vi "check_amp_mio.vi"() -> ()   [LabVIEW 2013]
uses:
  <vilib>/DAQmx/write.llb/DAQmx Write (Digital Bool 1Line 1Point).vi
  <vilib>/DAQmx/create/channels.llb/DAQmx Create Channel (DO-Digital Output).vi
  <vilib>/DAQmx/miscellaneous.llb/DAQmx Fill In Error Info.vi
panel:
  in  "data":bool
  in  "lines":tag
  in  "Exit":bool
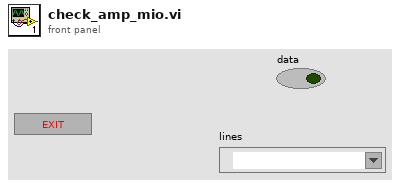
[diagram p1: front panel]
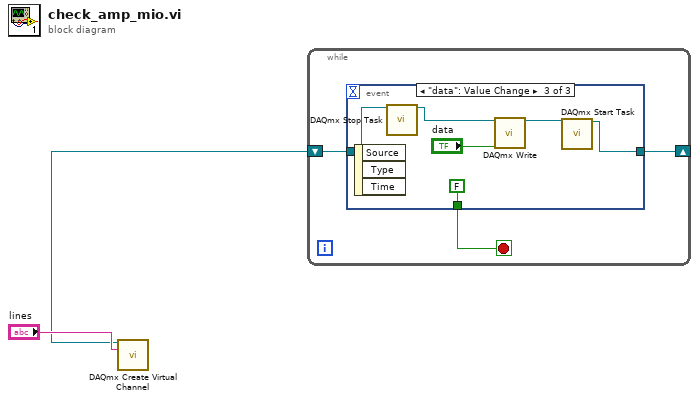
[diagram p0: block diagram]
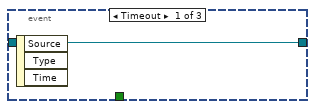
[diagram p2: hidden frame]
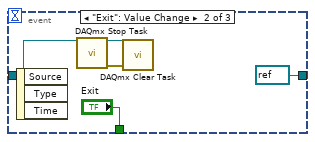
[diagram p3: hidden frame]
diagram:
  n1 = call-poly <vilib>:"DAQmx Create Virtual Channel.vi"("lines"="lines") -> ("task out"=w1:refnum<k21>)  [unwired: 13 in, 1 out]
  n2 = while {
    shift-right: [w3] -> _
    shift-left: w1 -> [w5]
    stop <- w4 stop-if-true
    n3 = event shown="[2] \"data\": Value Change" {
      selector: _ -> [_ _ _]
      dyn-events: _ -> [_ _ _]
      timeout: _ -> [_ _ _]
      tunnel: w5 -> [w6 w11 w12]
      tunnel: [_ "Exit" FALSE ("Exit")] -> w4
      tunnel: [w6 refnum<k21> refnum ("task out") w16] -> w3
      event Timeout {
        n4 = event-data() -> ()  [unwired: 1 in, 3 out]
      }
      event "Exit": Value Change {
        n5 = event-data() -> ()  [unwired: 1 in, 3 out]
        n6 = call <vilib>:"DAQmx Stop Task.vi"("task/channels in"=w11) -> ("task out"=w9:refnum<k21>, "error out"=w8:errorcluster)  [unwired: 13 in]
        n7 = call <vilib>:"DAQmx Clear Task.vi"("task in"=w9, "error in"=w8) -> ()  [unwired: 13 in, 1 out]
      }
      event "data": Value Change {
        n8 = event-data() -> ()  [unwired: 1 in, 3 out]
        n9 = call <vilib>:"DAQmx Stop Task.vi"("task/channels in"=w12) -> ("task out"=w13:refnum<k21>)  [unwired: 13 in, 1 out]
        n10 = call-poly <vilib>:"DAQmx Write.vi"("task/channels in"=w13, "data"="data") -> ("task out"=w17:refnum<k21>)  [unwired: 11 in, 2 out]
        n11 = call <vilib>:"DAQmx Start Task.vi"("task/channels in"=w17) -> ("task out"=w16:refnum<k21>)  [unwired: 13 in, 1 out]
      }
    }
  }
